vi "Problema3_1.vi"() -> ()   [LabVIEW 2020]
panel:
  out "?":dbl[][](graph)
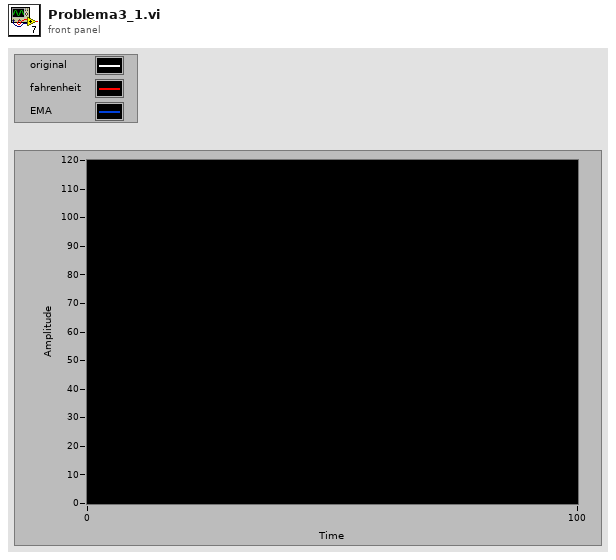
[diagram p1: front panel]
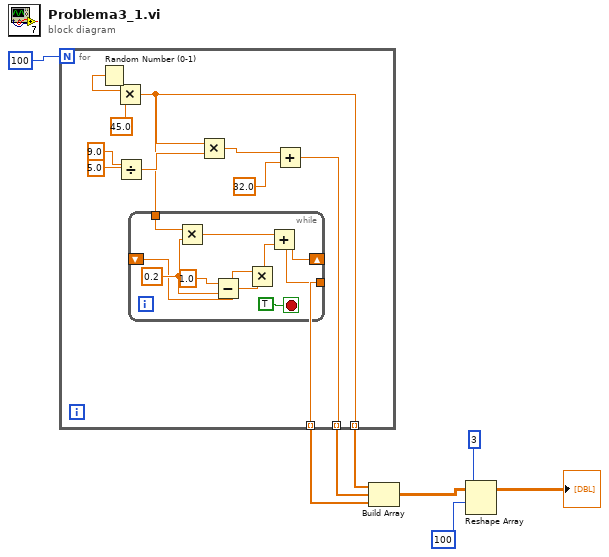
[diagram p0: block diagram]
diagram:
  n1 = for {
    N: 100 -> [_]
    tunnel: [w11] -> w5 mode=indexing
    tunnel: [w10] -> w4 mode=indexing
    tunnel: [w9] -> w3 mode=indexing
    n2 = Random Number (0-1)() -> (number: 0 to 1=w18:dbl)
    n3 = Multiply(x=w18, y=45.0) -> (x*y=w11:dbl)
    n4 = Divide(x=9.0, y=5.0) -> (x/y=w14:dbl)
    n5 = while {
      shift-right: [w19] -> _
      shift-left: _ -> [w21]
      tunnel: w11 -> [w25]
      tunnel: [w19] -> w9
      stop <- TRUE stop-if-true
      w23 = 0.2 ("y")
      n6 = Multiply(x=w25, y=w23) -> (x*y=w26:dbl)
      n7 = Subtract(x=1.0, y=w23) -> (x-y=w22:dbl)
      n8 = Multiply(x=w21, y=w22) -> (x*y=w20:dbl)
      n9 = Add(x=w26, y=w20) -> (x+y=w19:dbl)
    }
    n10 = Multiply(x=w11, y=w14) -> (x*y=w15:dbl)
    n11 = Add(x=w15, y=32.0) -> (x+y=w10:dbl)
  }
  n12 = Build Array(w5, w4, w3) -> (w2:dbl[][])
  n13 = Reshape Array(w2, 100 ("dimension size"), 3 ("dimension size")) -> (→"?":dbl[][])
